vi "Get SPI Engine Commands 128-bit.vi"(6 "Ready for Output":bool, 8 "error in":errorcluster, 11 "SPI Engine Resources":T5={"To SPI Engine Data FIFO"="DLU To SPI Engine Data FIFO", "From SPI Engine Data FIFO"="SPI Engine to DLU Data FIFO", "Data to SPI Engine Cache Register"="Data to SPI Engine (Cache)", "SPI Transaction Settings Cache Register"="SPI PHY Settings to SPI Engine (Cache)"}) -> (0 "error out":errorcluster, 1 "Output Valid":bool, 2 "SPI Transaction Packet":T1={"Start Strobe"=FALSE, "SPI Data"=[FALSE, FALSE, FALSE, FALSE, FALSE, FALSE, FALSE, FALSE, FALSE, FALSE, FALSE, FALSE, FALSE, FALSE, FALSE, FALSE, FALSE, FALSE, FALSE, FALSE, FALSE, FALSE, FALSE, FALSE, FALSE, FALSE, FALSE, FALSE, FALSE, FALSE, FALSE, FALSE, FALSE, FALSE, FALSE, FALSE, FALSE, FALSE, FALSE, FALSE, FALSE, FALSE, FALSE, FALSE, FALSE, FALSE, FALSE, FALSE, FALSE, FALSE, FALSE, FALSE, FALSE, FALSE, FALSE, FALSE, FALSE, FALSE, FALSE, FALSE, FALSE, FALSE, FALSE, FALSE, FALSE, FALSE, FALSE, FALSE, FALSE, FALSE, FALSE, FALSE, FALSE, FALSE, FALSE, FALSE, FALSE, FALSE, FALSE, FALSE, FALSE, FALSE, FALSE, FALSE, FALSE, FALSE, FALSE, FALSE, FALSE, FALSE, FALSE, FALSE, FALSE, FALSE, FALSE, FALSE, FALSE, FALSE, FALSE, FALSE, FALSE, FALSE, FALSE, FALSE, FALSE, FALSE, FALSE, FALSE, FALSE, FALSE, FALSE, FALSE, FALSE, FALSE, FALSE, FALSE, FALSE, FALSE, FALSE, FALSE, FALSE, FALSE, FALSE, FALSE, FALSE, FALSE, FALSE, FALSE], "SPI Settings"={"Chip Select ID"=0, "SPI Physical Settings"={"Divide Value"=0, "Transfer Length (bits)"=1, "CS Asserted Polarity"=FALSE, "Clock Polarity (CPOL)"=FALSE, "Clock Phase (CPHA)"=FALSE, "Lengthen MISO Setup"=FALSE, "Direction Change Bit"=0, "MOSI Starts as Output"=FALSE, "Tristatable MOSI"=FALSE}}} {"SPI Settings"."SPI Physical Settings"."Direction Change Bit" max=64 step=1; "SPI Settings"."SPI Physical Settings"."Transfer Length (bits)" min=1 max=64 step=1}, 3 "SPI Engine Resources":T5={"To SPI Engine Data FIFO"="DLU To SPI Engine Data FIFO", "From SPI Engine Data FIFO"="SPI Engine to DLU Data FIFO", "Data to SPI Engine Cache Register"="Data to SPI Engine (Cache)", "SPI Transaction Settings Cache Register"="SPI PHY Settings to SPI Engine (Cache)"}, 5 "Start Strobe":bool)   [LabVIEW 2015, in "SPI API.lvlib"]
uses:
  SPI API.lvlib
  Controls/SPI Engine Resources 128-bit.ctl
  Controls/SPI API Transaction Packet 128-bit.ctl
  Controls/SPI API Data 128-bit.ctl
  Controls/SPI Transaction Settings.ctl
  <userlib>/_NI SPI IP/FPGA/Controllers/Public/Transfer Settings.ctl
  Controls/SPI API Engine Receiver States.ctl
  SPI Engine.Get Commands.Read FIFO 128-bit.vi
  <userlib>/_NI SPI IP/FPGA/Controllers/NI SPI IP FPGA.lvlib
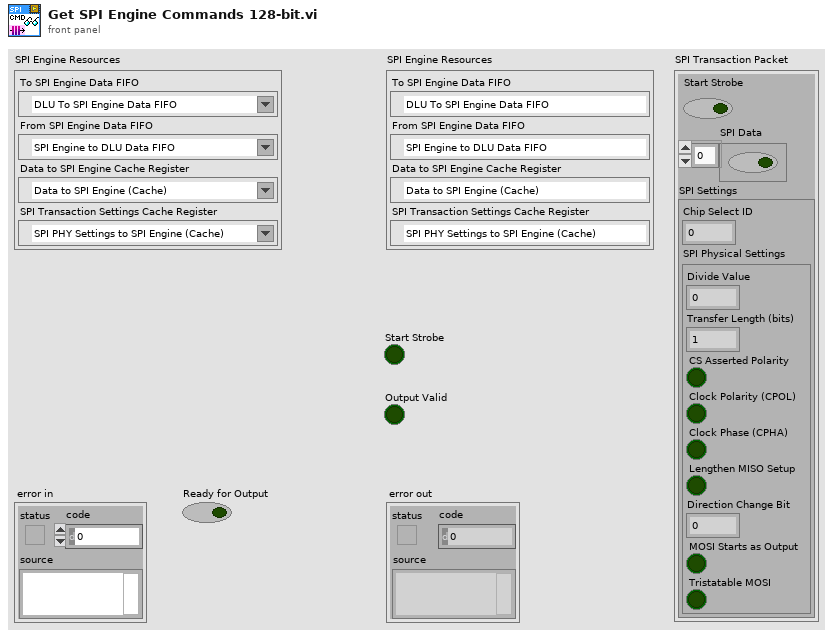
[diagram p1: front panel]
types:
  T1 = typedef "SPI API.lvlib/SPI API Transaction Packet 128-bit.ctl" = cluster{"Start Strobe":bool, "SPI Data":T2, "SPI Settings":T3}
  T2 = typedef "SPI API.lvlib/SPI API Data 128-bit.ctl" = bool[]
  T3 = typedef "SPI API.lvlib/SPI Transaction Settings.ctl" = cluster{"Chip Select ID":u8, "SPI Physical Settings":T4}
  T4 = typedef "NI SPI IP FPGA.lvlib/Transfer Settings.ctl" = cluster{"Divide Value":u8, "Transfer Length (bits)":u8, "CS Asserted Polarity":bool, "Clock Polarity (CPOL)":bool, "Clock Phase (CPHA)":bool, "Lengthen MISO Setup":bool, "Direction Change Bit":u8, "MOSI Starts as Output":bool, "Tristatable MOSI":bool}
  T5 = typedef "SPI API.lvlib/SPI Engine Resources 128-bit.ctl" = cluster{"To SPI Engine Data FIFO":refnum<k21>, "From SPI Engine Data FIFO":refnum<k21>, "Data to SPI Engine Cache Register":refnum<k21>, "SPI Transaction Settings Cache Register":refnum<k21>}
  T6 = typedef "SPI API.lvlib/SPI API Engine Receiver States.ctl" = enum16{"Wait for Start Command", "Deassert Start Probe"}
  T7 = typedef "SPI API.lvlib/SPI API Transmit Data 128-bit.ctl" = cluster{"SPI Data":T2, "SPI Settings":T3}
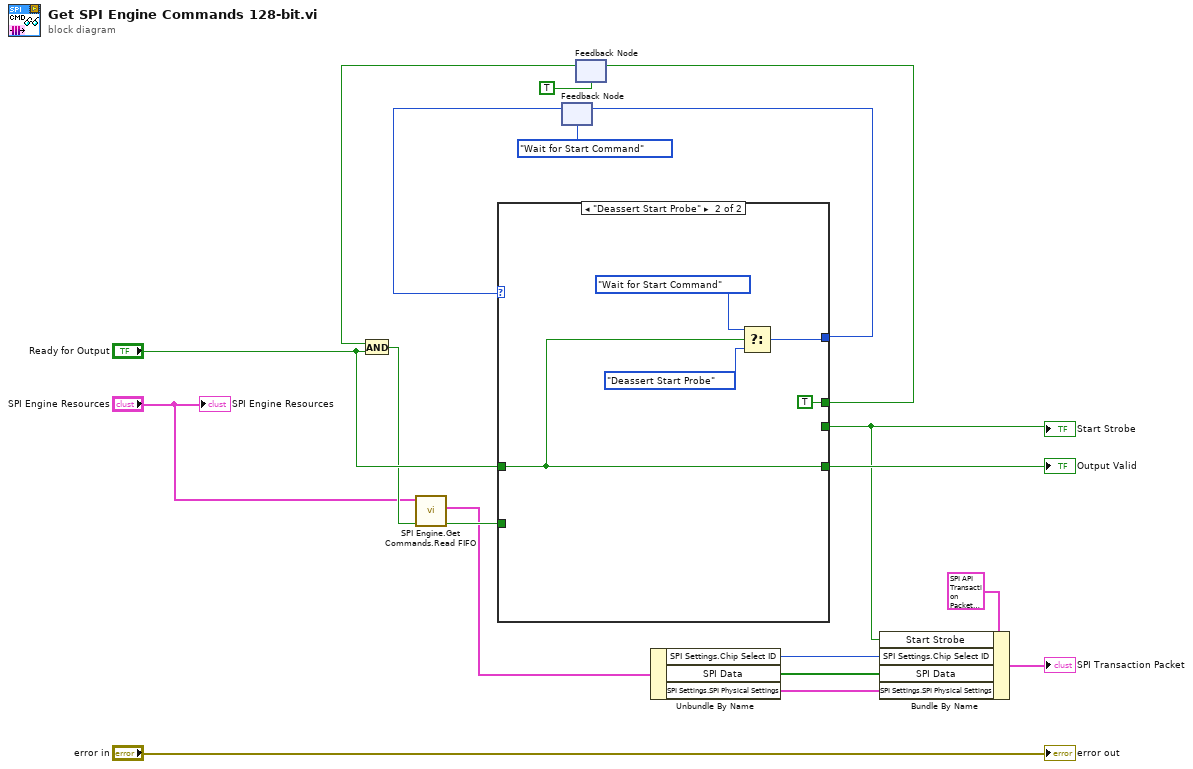
[diagram p0: block diagram]
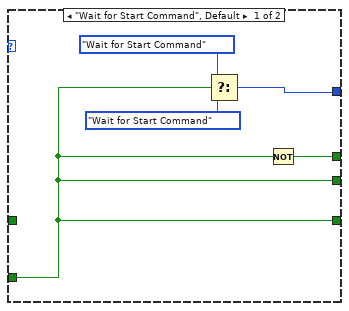
[diagram p2: hidden frame]
diagram:
  n1 = feedback #1(SPI_API_Engine_Receiver_States."Wait for Start Command") -> (w18:T6)
  n2 = feedback #2(TRUE) -> (w15:bool)
  n3 = And(x=w15, y="Ready for Output") -> (x .and. y?=w6:bool)
  n4 = call-poly "SPI Engine.Get Commands.Read FIFO.vi"("Get New Data"=w6, "SPI Engine Resources"="SPI Engine Resources") -> ("Output Valid"=w5:bool, "SPI Transaction Packet"=w1:T7)  [unwired: 7 in, 1 out]
  n5 = case shown="\"Deassert Start Probe\"" w18 {
    tunnel: [w22 w25] -> w17
    tunnel: [w21 TRUE] -> w16
    tunnel: w5 -> [w20 _]
    tunnel: [w20 _] -> w7
    tunnel: [w20 w27] -> w13
    tunnel: "Ready for Output" -> [_ w27]
    frame "Wait for Start Command", Default {
      n6 = Select(t=SPI_API_Engine_Receiver_States."Wait for Start Command", s=w20, f=SPI_API_Engine_Receiver_States."Wait for Start Command") -> (s? t:f=w22:T6)
      n7 = Not(x=w20) -> (.not. x?=w21:bool)
    }
    frame "Deassert Start Probe" {
      n8 = Select(t=SPI_API_Engine_Receiver_States."Wait for Start Command", s=w27, f=SPI_API_Engine_Receiver_States."Deassert Start Probe") -> (s? t:f=w25:T6)
    }
  }
  "Start Strobe" <- w7
  "Output Valid" <- w13
  n9 = feedback-in #1(w17) -> ()
  n10 = feedback-in #2(w16) -> ()
  n11 = Unbundle By Name(w1) -> ("SPI Settings.Chip Select ID"=w11:u8, "SPI Data"=w10:T2, "SPI Settings.SPI Physical Settings"=w9:T4)
  n12 = Bundle By Name(cluster=T1 {"Start Strobe"=FALSE, "SPI Data"=[FALSE, FALSE, FALSE, FALSE, FALSE, FALSE, FALSE, FALSE, FALSE, FALSE, FALSE, FALSE, FALSE, FALSE, FALSE, FALSE, FALSE, FALSE, FALSE, FALSE, FALSE, FALSE, FALSE, FALSE, FALSE, FALSE, FALSE, FALSE, FALSE, FALSE, FALSE, FALSE, FALSE, FALSE, FALSE, FALSE, FALSE, FALSE, FALSE, FALSE, FALSE, FALSE, FALSE, FALSE, FALSE, FALSE, FALSE, FALSE, FALSE, FALSE, FALSE, FALSE, FALSE, FALSE, FALSE, FALSE, FALSE, FALSE, FALSE, FALSE, FALSE, FALSE, FALSE, FALSE, FALSE, FALSE, FALSE, FALSE, FALSE, FALSE, FALSE, FALSE, FALSE, FALSE, FALSE, FALSE, FALSE, FALSE, FALSE, FALSE, FALSE, FALSE, FALSE, FALSE, FALSE, FALSE, FALSE, FALSE, FALSE, FALSE, FALSE, FALSE, FALSE, FALSE, FALSE, FALSE, FALSE, FALSE, FALSE, FALSE, FALSE, FALSE, FALSE, FALSE, FALSE, FALSE, FALSE, FALSE, FALSE, FALSE, FALSE, FALSE, FALSE, FALSE, FALSE, FALSE, FALSE, FALSE, FALSE, FALSE, FALSE, FALSE, FALSE, FALSE, FALSE, FALSE, FALSE, FALSE], "SPI Settings"={"Chip Select ID"=0, "SPI Physical Settings"={"Divide Value"=0, "Transfer Length (bits)"=1, "CS Asserted Polarity"=FALSE, "Clock Polarity (CPOL)"=FALSE, "Clock Phase (CPHA)"=FALSE, "Lengthen MISO Setup"=FALSE, "Direction Change Bit"=0, "MOSI Starts as Output"=FALSE, "Tristatable MOSI"=FALSE}}} ("SPI Transaction Packet"), "Start Strobe"=w7, "SPI Settings.Chip Select ID"=w11, "SPI Data"=w10, "SPI Settings.SPI Physical Settings"=w9) -> (→"SPI Transaction Packet":T1)
  "error out" <- "error in"
  "SPI Engine Resources" <- "SPI Engine Resources"
